vi "readdata_830.vi"(2 "error in":errorcluster, 3 "Command":string="outp ? 1", 4 "timeout":i32=300, 5 "Lockin Address":string="12") -> (0 "error out":errorcluster, 1 "Data":dbl format="%#.3p")   [LabVIEW 2010]
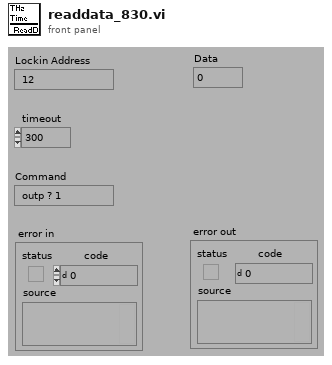
[diagram p1: front panel]
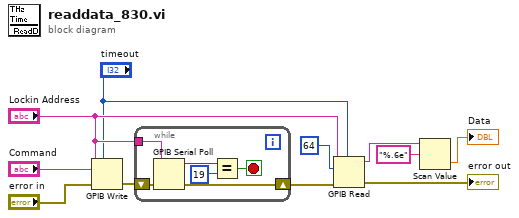
[diagram p0: block diagram]
diagram:
  n1 = GPIB Write(0:"Lockin Address", 1:"Command", 3:"error in", 4:"timeout") -> (6:w10:errorcluster)  [unwired: 1 in, 1 out]
  n2 = while {
    shift-left: w10 -> [w15]
    shift-right: [w14] -> w11
    tunnel: "Lockin Address" -> [w12]
    stop <- w16 stop-if-true
    n3 = GPIB Serial Poll(0:w12, 1:w15) -> (2:w13:i16, 4:w14:errorcluster)  [unwired: 1 out]
    n4 = Equal?(x=w13, y=19) -> (x = y?=w16:bool)
  }
  n5 = GPIB Read(0:"Lockin Address", 1:64, 3:w11, 4:"timeout") -> (5:w5:string, 7:→"error out":errorcluster)  [unwired: 1 in, 1 out]
  n6 = Scan Value(string=w5, format string="%.6e") -> (value=→"Data":dbl)  [unwired: 1 in, 1 out]
